vi "INIT Add Database.vi"(8 "error in (no error)":errorcluster, 10 "DB Alias data":T1, 11 "Device Item Ref in":T2 format="%.0x") -> (0 "error out":errorcluster, 3 "Device Item Ref out":T2 format="%.0x")   [LabVIEW 2018, in "CAN Gateway System Explorer.lvlib"]
uses:
  CAN Gateway System Explorer.lvlib
  <vilib>/NI Veristand/Custom Device API/Custom Device Item Ref.ctl
  Types/Alias DB data.ctl
  Shared/Constants.vi
  <vilib>/NI Veristand/Custom Device Tools/Custom Device Utility Library/NI VeriStand - Search for Item by GUID.vi
  <vilib>/NI Veristand/Custom Device Tools/Custom Device Utility Library/NI VeriStand - Search for Item by Name.vi
  <vilib>/NI Veristand/Custom Device Tools/Custom Device Utility Library/Custom Device Utility Library.lvlib
  Shared/CAN Gateway Shared.lvlib
  <vilib>/NI Veristand/Custom Device API/Custom Device API.lvlib
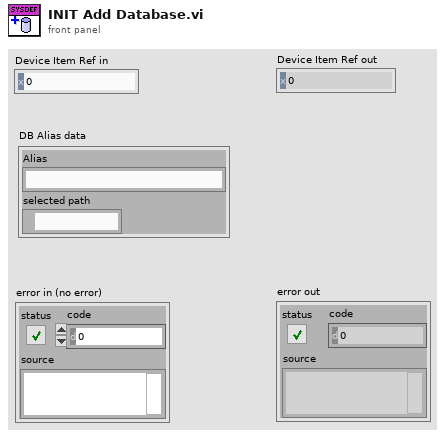
[diagram p1: front panel]
types:
  T1 = typedef "CAN Gateway System Explorer.lvlib/Alias DB data.ctl" = cluster{"Alias":string, "selected path":path}
  T2 = typedef "Custom Device API.lvlib/Custom Device Item Ref.ctl" = u64
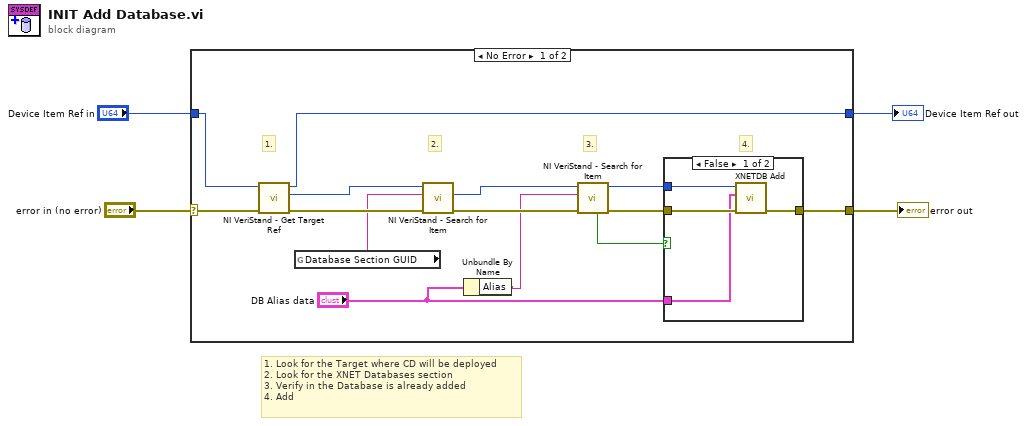
[diagram p0: block diagram]
diagram:
  # "1. Look for the Target where CD will be deployed\n2. Look for the XNET Databases section\n3. Verify in the Database is already added\n4. Add"
  n1 = case shown="No Error" "error in (no error)" {
    selector: "error in (no error)" -> [w18 w24]
    tunnel: "Device Item Ref in" -> [w15 w25]
    tunnel: [w9 w25] -> w2
    tunnel: [w8 w24] -> w1
    frame No Error {
      # "4."
      # "3."
      # "2."
      # "1."
      n2 = call <vilib>:"NI VeriStand - Get Target Ref.vi"("error in"=w18, "Item Ref in"=w15) -> ("error out"=w17:errorcluster, "Target Ref"=w10:T2, "Item Ref out"=w9:T2)  [unwired: 6 in, 1 out]
      n3 = global read "Constants.vi" "Database Section GUID"() -> (w5:string)
      n4 = call-poly <vilib>:"NI VeriStand - Search for Item.vi"("error in"=w17, "Item GUID"=w5, "Section Ref in"=w10) -> ("error out"=w14:errorcluster, "Item Ref"=w16:T2)  [unwired: 5 in, 2 out]
      n5 = Unbundle By Name("DB Alias data") -> ("Alias"=w6:string)
      n6 = call-poly <vilib>:"NI VeriStand - Search for Item.vi"("error in"=w14, "Item Name"=w6, "Section Ref in"=w16) -> ("error out"=w12:errorcluster, "Section Ref out"=w11:T2, "Found"=w13:bool)  [unwired: 5 in, 1 out]
      n7 = case shown="False" w13 {
        tunnel: w12 -> [w22 w23]
        tunnel: [w21 w23] -> w8
        tunnel: w11 -> [w20 _]
        tunnel: "DB Alias data" -> [w19 _]
        frame False {
          n8 = call "XNETDB Add.vi"("error in (no error)"=w22, "DB Alias data"=w19, "Databases Section Ref"=w20) -> ("error out"=w21:errorcluster)  [unwired: 8 in]
        }
        frame True {
        }
      }
    }
    frame Error {
    }
  }
  "error out" <- w1
  "Device Item Ref out" <- w2
